vi "Read LLP Packets From Host.vi"(2 "llp packets dma fifo":refnum<k21>, 12 "ready for output":bool=TRUE) -> (4 "dram word":T1, 10 "output valid":bool)   [LabVIEW 2020, in "GettingStarted_Gen_148X_FPGA.lvlib"]
uses:
  GettingStarted_Gen_148X_FPGA.lvlib
  <instrlib>/_niInstr/Memory/v1/FPGA/Memory/Public/U256.ctl
  <vilib>/rvi/DataTransferAndStorage/Container/Common/niFpgaContainerExecOnDevCompGetState.vi
  <vilib>/rvi/Emulation/niFpgaSctlEmulationGetInTimedLoop.vi
  <vilib>/rvi/errors/niFpgaSetErrorForExecOnDevCompSimple.vi
  <vilib>/rvi/eio/common/nirviEmuReportErrorAndStop.vi
  <vilib>/rvi/interface/RandomDataEmulation/nirviRandomDataAcquireLock.vi
  <vilib>/rvi/interface/RandomDataEmulation/nirviRandomDataQueueStore.vi
  <vilib>/rvi/interface/RandomDataEmulation/nirviRandomDataReleaseLock.vi
  <vilib>/rvi/interface/RandomDataEmulation/nirviFPGAContextMergeError.vi
  <vilib>/rvi/interface/RandomDataEmulation/nirviRandomDataCheckExitLoopConditions.vi
  <vilib>/express/rvi/timingcommon/nirviCommon.vi
  <vilib>/rvi/interface/RandomDataEmulation/niFpgaRandomDataHandleErrors.vi
  <instrlib>/_niInstr/Data Formatting/v1/FPGA/Private/Convert/U8 array to Boolean Array.vi
  <vilib>/rvi/DataTransferAndStorage/Container/XNode/niFpgaContainer.xnode
  <vilib>/rvi/FIFO/Fifo_Resource/niFpgaFifoEmulationRefInMultiElement.vi
  <instrlib>/_niInstr/Data Formatting/v1/FPGA/niInstr Data Formatting v1 FPGA.lvlib
  <instrlib>/_niInstr/Memory/v1/FPGA/Memory/niInstr Memory v1 FPGA.lvclass
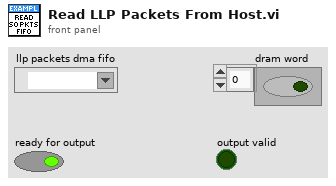
[diagram p1: front panel]
types:
  T1 = typedef "niInstr Memory v1 FPGA.lvclass/U256.ctl" = bool[]
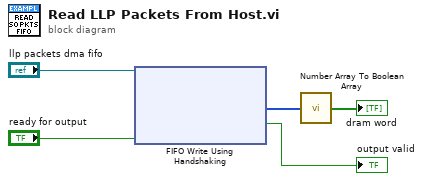
[diagram p0: block diagram]
diagram:
  n1 = xnode ("FIFO Write Using Handshaking")("Ready for Output"="ready for output", "FIFO In"="llp packets dma fifo") -> ("Element"=w4:u8[], "Output Valid"=→"output valid":bool)  [unwired: 1 out]
  n2 = call-poly <instrlib>:"Number Array To Boolean Array.vi"("data in"=w4) -> ("data out"=→"dram word":bool[])  [unwired: 14 in]
